vi "Decorate.vi"(10 "Actor":refnum<class "Actor.lvclass">, 11 "TEMPLATE Actor in":refnum<class "TEMPLATE Actor.lvclass">) -> (3 "TEMPLATE Actor out":refnum<class "TEMPLATE Actor.lvclass">)   [LabVIEW 2020, in "_Template.lvlib" / "Templates.lvlib" / "TEMPLATE Actor.lvlib" / "TEMPLATE Actor.lvclass"]
uses:
  TEMPLATE Actor.lvclass
  jettl/jettl/Actor/Actor/Actor.lvclass
  TEMPLATE Actor.lvclass/TEMPLATE Actor.ctl
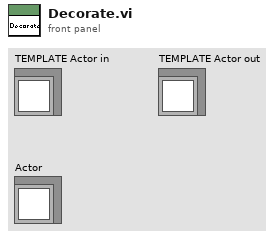
[diagram p1: front panel]
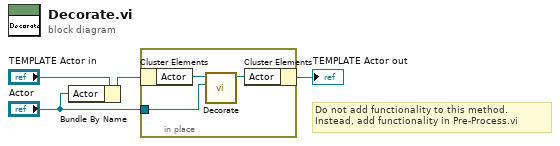
[diagram p0: block diagram]
diagram:
  # "Do not add functionality to this method. Instead, add functionality in Pre-Process.vi"
  n1 = Bundle By Name(cluster="TEMPLATE Actor in", "Actor"="Actor") -> (w3:refnum<class "TEMPLATE Actor.lvclass">)
  n2 = in-place {
    in-place-border: "Actor" -> [w5]
    n3 = in-place-cluster #1(w3) -> ("Actor"=w7:refnum<class "Actor.lvclass">)
    n4 = call-dynamic "Decorate.vi"("Actor"=w5, "Actor in"=w7) -> ("Actor out"=w6:refnum<class "Actor.lvclass">)  [unwired: 9 in]
    n5 = in-place-cluster #1("Actor"=w6) -> (→"TEMPLATE Actor out":refnum<class "TEMPLATE Actor.lvclass">)
  }
